vi "v_limiter.vi"(7 "Parameters":T2={"Stimulus"={"Type"=enum."Off", "Phase"=0.0, "Amplitude"=[], "Injection point"=enum."Total pose", "Closed loop"=FALSE, "Offset"=[], "Tip -> world"=FALSE, "Frequency"=0.0, "Length"=0.0}, "Goal Filter A"={"Speedup max"=0.0, "Speedup thresh"=0.0, "Speedup nonlin"=0.0, "Filters"=[]}, "Mode controls"={"Hold"=FALSE, "Cancellation"=FALSE, "Goal filter"=FALSE, "Trigger"=FALSE}, "Manipulator type"=enum."Current piezo", "Manipulator calibration"={"Tool offsets"=[[0.0, 0.0, 36200.0]], "Handle light calibration"=[], "Base pivots"=[], "Output pivots"=[], "Length center"=0.0, "Workspace height"=[], "Workspace diameter"=[0.0, 0.0, 36200.0], "Stack travel"=400.0, "Saturation pos"=375.0, "Inverse filters"=[], "Strut length"=0.0}, "Network"={"Remote Host"="", "Send Status"=FALSE, "Send Port"=0, "Recv Commands"=FALSE, "Recv Port"=0}, "Goal Filter B"={"Speedup max"=0.0, "Speedup thresh"=0.0, "Speedup nonlin"=0.0, "Filters"=[]}, "Cancellation"={"KP"={"XY"=0.0, "Rxy"=0.0, "Z"=0.0, "Rz"=0.0}, "KI"=0.0, "KD"={"XY"=0.0, "Rxy"=0.0, "Z"=0.0, "Rz"=0.0}, "Max vel"=20.0, "Max acc"=0.001, "Int error limit"=3.0, "RCM gain"=0.0, "Bypass"=FALSE, "Degraded gain"=0.0}, "Transition time"=0.0, "Estimation"={"Link"={"Measure noise"=[], "Process noise"=[], "Alt process noise"=[], "Alt turnoff cycles"=20, "Innovation limit"=[], "Residue threshold"=0.0, "Enable"=FALSE}, "Handle"={"Measure noise"=[], "Process noise"=[], "State limits"=[], "Innovation limit"=[], "Prediction Lookahead"=0.0, "Enable"=FALSE}}} {"Transition time" format="%_3f"; "Cancellation"."Degraded gain" min=0 max=1 step=0.1 format="%#_3p"; "Cancellation"."RCM gain" min=0 max=1 step=0.1 format="%#_3p"; "Cancellation"."KD"."Rz" min=-1 max=1 step=0.01 format="%#_3p"; "Cancellation"."KD"."Rxy" min=-1 max=1 step=0.01 format="%#_3p"; "Cancellation"."KD"."Z" min=-1 max=1 step=0.01 format="%#_3p"; "Cancellation"."KD"."XY" min=-1 max=1 step=0.01 format="%#_3p"; "Cancellation"."KI" min=0 max=1 step=0.01 format="%#_3p"; "Cancellation"."KP"."Rz" min=-1 max=1 step=0.01 format="%#_3p"; "Cancellation"."KP"."Rxy" min=-1 max=1 step=0.01 format="%#_3p"; "Cancellation"."KP"."Z" min=-1 max=1 step=0.01 format="%#_3p"; "Cancellation"."KP"."XY" min=-1 max=1 step=0.01 format="%#_3p"; "Cancellation"."Max acc" format="%#_3p"; "Goal Filter B"."Filters"."V limit range" format="%_3p"; "Goal Filter B"."Filters"."V limit" format="%_3p"; "Goal Filter B"."Filters"."Upper Q" format="%_3f"; "Goal Filter B"."Filters"."Upper Fc" format="%_3p"; "Goal Filter B"."Filters"."Lower Q" format="%_3f"; "Goal Filter B"."Filters"."Scale factor" format="%_3f"; "Goal Filter B"."Filters"."Lower Fc" format="%_3p"; "Goal Filter B"."Speedup nonlin" format="%_3p"; "Goal Filter B"."Speedup thresh" format="%_3p"; "Goal Filter B"."Speedup max" format="%_3p"; "Manipulator calibration"."Strut length" format="%#_4p"; "Manipulator calibration"."Saturation pos" format="%#.1f"; "Manipulator calibration"."Stack travel" format="%#.1f"; "Manipulator calibration"."Length center" format="%#_4p"; "Manipulator calibration"."Output pivots" format="%#_6f"; "Manipulator calibration"."Base pivots" format="%#_6f"; "Manipulator calibration"."Handle light calibration" format="%#.1f"; "Goal Filter A"."Filters"."V limit range" format="%_3p"; "Goal Filter A"."Filters"."V limit" format="%_3p"; "Goal Filter A"."Filters"."Upper Q" format="%_3f"; "Goal Filter A"."Filters"."Upper Fc" format="%_3p"; "Goal Filter A"."Filters"."Lower Q" format="%_3f"; "Goal Filter A"."Filters"."Scale factor" format="%_3f"; "Goal Filter A"."Filters"."Lower Fc" format="%_3p"; "Goal Filter A"."Speedup nonlin" format="%_3p"; "Goal Filter A"."Speedup thresh" format="%_3p"; "Goal Filter A"."Speedup max" format="%_3p"; "Stimulus"."Length" min=0.0 max=100.0 step=100.0 format="%#_4p"; "Stimulus"."Frequency" min=0.0 step=100.0 format="%#_4g"; "Stimulus"."Offset" format="%#_3p"; "Stimulus"."Amplitude" format="%#_3p"; "Stimulus"."Phase" min=-180.0 max=360.0 step=100.0 format="%#.2f"}, 8 "Reset":bool, 9 "Sampling frequency":sgl=1.0 format="%0.2f", 10 "Goal position in":sgl[](array[numeric]), 11 "Goal filter":T1={"Lower Fc"=0.08, "Lower Q"=0.606, "Scale factor"=3.0, "Upper Fc"=2.0, "Upper Q"=0.606, "V limit"=1.5, "V limit range"=25.0} {"V limit range" format="%_3p"; "V limit" format="%_3p"; "Upper Q" format="%_3f"; "Upper Fc" format="%_3p"; "Lower Q" format="%_3f"; "Scale factor" format="%_3f"; "Lower Fc" format="%_3p"}) -> (1 "Goal position out":sgl[](array[numeric]), 4 "V limiting":bool)   [LabVIEW 2014]
uses:
  testing/Micron params.ctl
  testing/stimulus.ctl
  testing/injection_point.ctl
  goal_loop_parms.ctl
  testing/mode_conrols.ctl
  testing/manipulator_cal.ctl
  asap/labview/testing/probe_calibration.ctl
  host/network_params.ctl
  cancellation/sq_control_params.ctl
  cancellation/decoupled_gain.ctl
  cancellation/estimation_controls.ctl
  goal_filter_parms.ctl
  utilities/labview/norm_vec_single.vi
panel:
  # "Locals:"
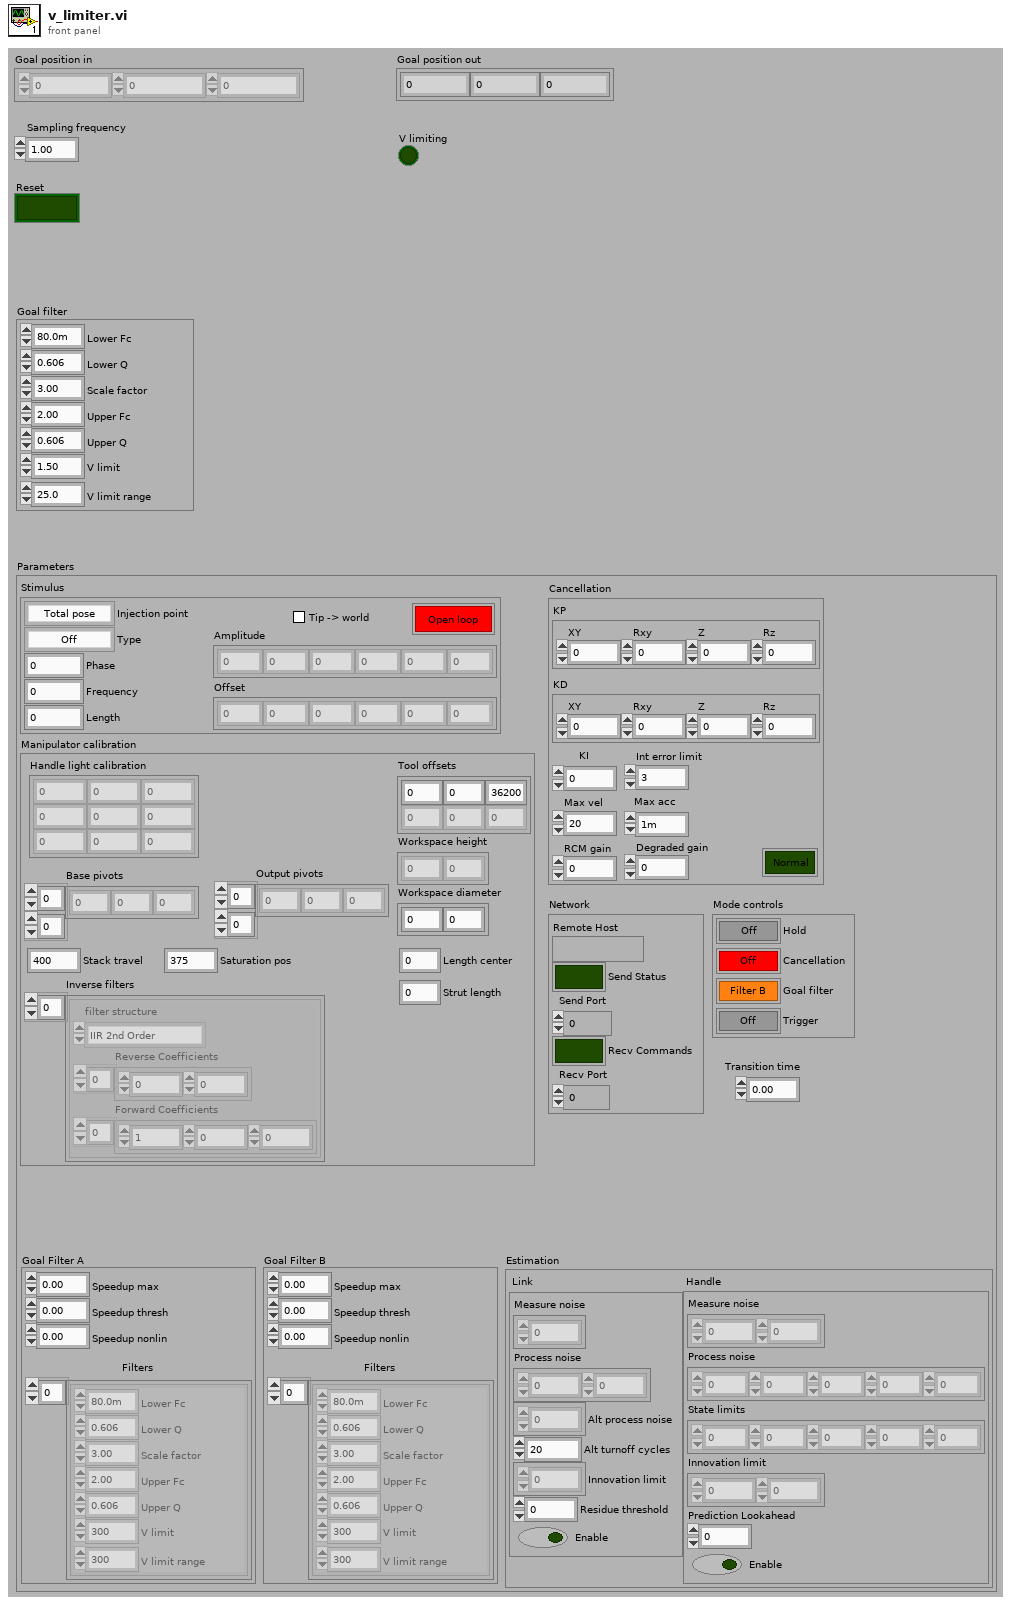
[diagram p1: front panel]
types:
  T1 = typedef "goal_filter_parms.ctl" = cluster{"Lower Fc":sgl, "Lower Q":sgl, "Scale factor":sgl, "Upper Fc":sgl, "Upper Q":sgl, "V limit":sgl, "V limit range":sgl}
  T2 = typedef "Micron params.ctl" = cluster{"Stimulus":T3, "Goal Filter A":T5, "Mode controls":T6, "Manipulator type":enum16{"Current piezo", "Voltage piezo"}, "Manipulator calibration":T7, "Network":T9, "Goal Filter B":T5, "Cancellation":T10, "Transition time":sgl, "Estimation":T12}
  T3 = typedef "stimulus.ctl" = cluster{"Type":enum16{"Off", "Step", "Sine", "Triangle", "Arbitrary"}, "Phase":dbl, "Amplitude":sgl[], "Injection point":T4, "Closed loop":bool, "Offset":sgl[], "Tip -> world":bool, "Frequency":dbl, "Length":dbl}
  T4 = typedef "injection_point.ctl" = enum16{"Total pose", "V limiter", "Goal ", "Link position", "KF link position", "Inverse kin", "Link goal", "Link error", "Controller", "Output", "Drive", "Light"}
  T5 = typedef "goal_loop_parms.ctl" = cluster{"Speedup max":sgl, "Speedup thresh":sgl, "Speedup nonlin":sgl, "Filters":cluster{"Lower Fc":sgl, "Lower Q":sgl, "Scale factor":sgl, "Upper Fc":sgl, "Upper Q":sgl, "V limit":sgl, "V limit range":sgl}[]}
  T6 = typedef "mode_conrols.ctl" = cluster{"Hold":bool, "Cancellation":bool, "Goal filter":bool, "Trigger":bool}
  T7 = typedef "manipulator_cal.ctl" = cluster{"Tool offsets":sgl[][], "Handle light calibration":T8, "Base pivots":sgl[][], "Output pivots":sgl[][], "Length center":sgl, "Workspace height":sgl[], "Workspace diameter":sgl[], "Stack travel":sgl, "Saturation pos":sgl, "Inverse filters":cluster{"filter structure":enum32{"IIR 2nd Order", "IIR 4th Order"}, "Reverse Coefficients":dbl[], "Forward Coefficients":dbl[]}[], "Strut length":sgl}
  T8 = typedef "probe_calibration.ctl" = sgl[][]
  T9 = typedef "network_params.ctl" = cluster{"Remote Host":string, "Send Status":bool, "Send Port":u16, "Recv Commands":bool, "Recv Port":u16}
  T10 = typedef "sq_control_params.ctl" = cluster{"KP":T11, "KI":sgl, "KD":T11, "Max vel":sgl, "Max acc":sgl, "Int error limit":sgl, "RCM gain":sgl, "Bypass":bool, "Degraded gain":sgl}
  T11 = typedef "decoupled_gain.ctl" = cluster{"XY":sgl, "Rxy":sgl, "Z":sgl, "Rz":sgl}
  T12 = typedef "estimation_controls.ctl" = cluster{"Link":cluster{"Measure noise":dbl[], "Process noise":dbl[], "Alt process noise":dbl[], "Alt turnoff cycles":i32, "Innovation limit":dbl[], "Residue threshold":dbl, "Enable":bool}, "Handle":cluster{"Measure noise":dbl[], "Process noise":dbl[], "State limits":dbl[], "Innovation limit":dbl[], "Prediction Lookahead":sgl, "Enable":bool}}
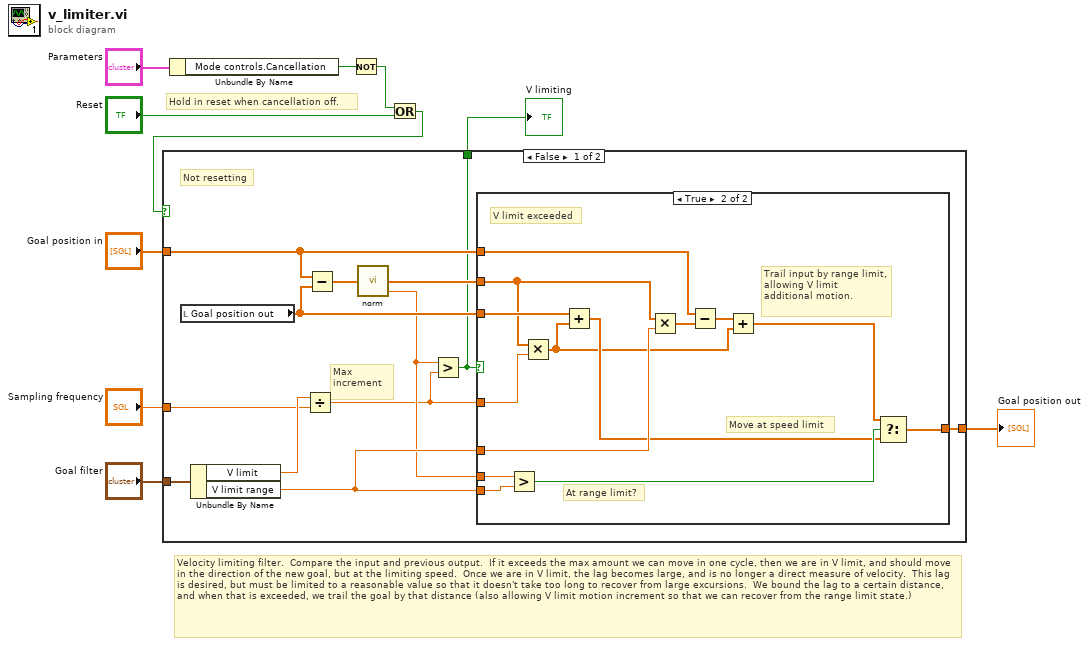
[diagram p0: block diagram]
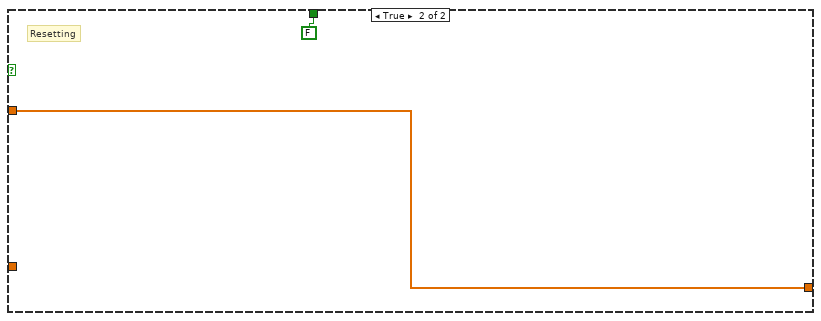
[diagram p3: hidden frame]
diagram:
  # "Velocity limiting filter.  Compare the input and previous output.  If it exceeds the max amount we can move in one cycle, then we are in V limit, and should move in the direction of the new goal, but at the limiting speed.  Once we are in V limit, the lag becomes large, and is no longer a direct measure of velocity.  This lag is desired, but must be limited to a reasonable value so that it doesn't take too long to recover from large excursions.  We bound the lag to a certain distance, and when that is exceeded, we trail the goal by that distance (also allowing V limit motion increment so that we can recover from the range limit state.)"
  # "Hold in reset when cancellation off."
  n1 = Unbundle By Name("Parameters") -> ("Mode controls.Cancellation"=w8:bool)
  n2 = Not(x=w8) -> (.not. x?=w9:bool)
  n3 = Or(x=w9, y="Reset") -> (x .or. y?=w6:bool)
  n4 = case shown="False" w6 {
    tunnel: "Goal position in" -> [w18 w39]
    tunnel: [w20 w39] -> w4
    tunnel: "Goal filter" -> [w22 _]
    tunnel: "Sampling frequency" -> [w14 _]
    tunnel: [w11 FALSE] -> w1
    frame False {
      # "Max increment"
      # "Not resetting"
      n5 = local read "Goal position out"() -> (w17:sgl[])
      n6 = Unbundle By Name(w22) -> ("V limit"=w15:sgl, "V limit range"=w16:sgl)
      n7 = Divide(x=w15, y=w14) -> (x/y=w12:sgl)
      n8 = Subtract(x=w18, y=w17) -> (x-y=w21:sgl[])
      n9 = call-poly "norm.vi"("vector"=w21) -> ("magnitude"=w13:sgl, "normalized vector"=w19:sgl[])  [unwired: 3 out]
      n10 = Greater?(x=w13, y=w12) -> (0:w11:bool)
      n11 = case shown="True" w11 {
        tunnel: [w23 w25] -> w20
        tunnel: w18 -> [w23 w34]
        tunnel: w13 -> [_ w36]
        tunnel: w16 -> [_ w37]
        tunnel: w19 -> [_ w33]
        tunnel: w17 -> [_ w35]
        tunnel: w16 -> [_ w32]
        tunnel: w12 -> [_ w24]
        frame False {
          # "V limit not exceeded"
        }
        frame True {
          # "Move at speed limit"
          # "Trail input by range limit, allowing V limit additional motion."
          # "V limit exceeded"
          # "At range limit?"
          n12 = Greater?(x=w36, y=w37) -> (0:w30:bool)
          n13 = Multiply(x=w33, y=w24) -> (x*y=w27:sgl[])
          n14 = Add(x=w35, y=w27) -> (x+y=w29:sgl[])
          n15 = Multiply(x=w33, y=w32) -> (x*y=w31:sgl[])
          n16 = Subtract(x=w34, y=w31) -> (x-y=w28:sgl[])
          n17 = Add(x=w28, y=w27) -> (x+y=w26:sgl[])
          n18 = Select(t=w26, s=w30, f=w29) -> (s? t:f=w25:sgl[])
        }
      }
    }
    frame True {
      # "Resetting"
    }
  }
  "Goal position out" <- w4
  "V limiting" <- w1
